vi "Launch Actors Wrapper.vi"() -> ()   [LabVIEW 2020]
uses:
  User Forms/TRExpRaw/TRExperimentsRaw.lvclass
  C:/Users/User/Desktop/Raman Program/Database OOP/source/Forms AF/Forms Controller/Form Controller/Panel Form Controller.lvclass
  Database OOP/Database Libraries/ADODB/ADODB Class/ADODB.lvclass
  C:/Users/User/Desktop/Raman Program/Database OOP/source/Database OOP/Database Libraries/Database Interfaces/Database Advanced Schema Class/Database Adv Schema.lvclass
  Database OOP/Database Libraries/ADODB/UDL Connection Class/UDL Connection.lvclass
  C:/Users/User/Desktop/Raman Program/Database OOP/source/Database OOP/Database Libraries/Database Interfaces/Database Connection Class/Database Connection.lvclass
  Forms Server/Form Server Wrapper/Form Server Wrapper.lvclass
  Database OOP/Table Libraries/Basic Table/Basic Table Class/Basic Table.lvclass
panel:
  in  "stop":bool
  out "Table Control":string[][](table)
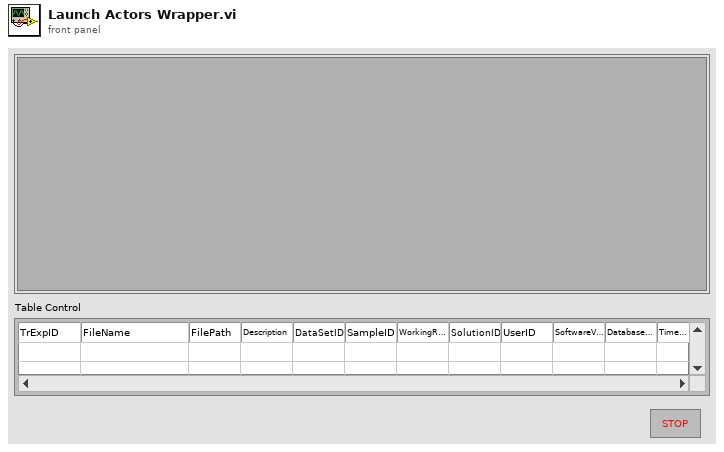
[diagram p1: front panel]
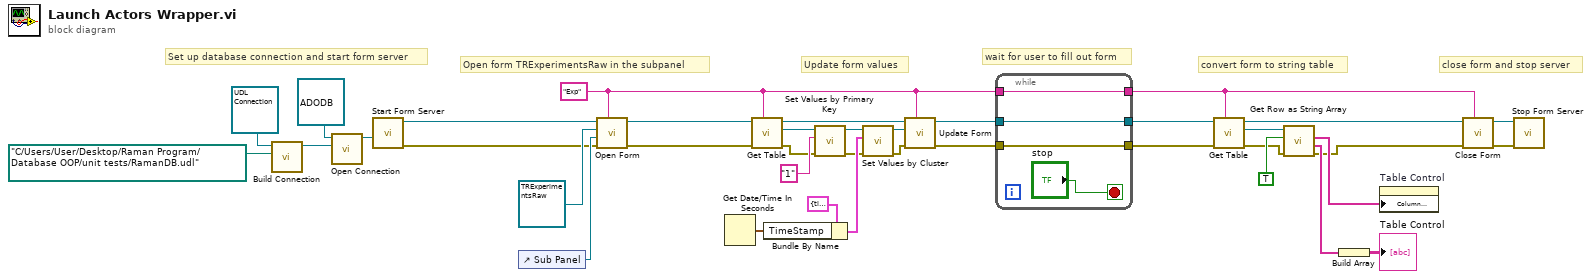
[diagram p0: block diagram]
diagram:
  w16 = "Exp" ("Name")
  # "close form and stop server"
  # "convert form to string table"
  # "wait for user to fill out form"
  # "Update form values"
  # "Open form TRExperimentsRaw in the subpanel"
  # "Set up database connection and start form server"
  n1 = call "Build Connection.vi"("*.udl file path"=path "C:/Users/User/Desktop/Raman Program/Database OOP/unit tests/RamanDB.udl", "UDL Connection in"=refnum<class "UDL Connection.lvclass"> refnum) -> ("UDL Connection out"=w27:refnum<class "UDL Connection.lvclass">)  [unwired: 8 in, 1 out]
  n2 = call-dynamic "Open Connection.vi"("Connection"=w27, "ADODB in"=refnum<class "ADODB.lvclass"> refnum ("ADODB.lvlib:ADODB.lvclass")) -> ("ADODB out"=w25:refnum<class "ADODB.lvclass">)  [unwired: 8 in, 1 out]
  n3 = call "Start Form Server.vi"("Database"=w25) -> ("error out"=w35:errorcluster, "Form Server Wrapper out"=w36:refnum<class "Form Server Wrapper.lvclass">)  [unwired: 9 in]
  n4 = control-ref of="Sub Panel"() -> (w38:refnum<vi>)
  n5 = call "Open Form.vi"("Name"=w16, "error in (no error)"=w35, "Sub Panel Refnum"=w38, "Form"=refnum<class "TRExperimentsRaw.lvclass"> refnum ("Forms.lvlib:TRExperimentsRaw.lvclass"), "Form Server Wrapper in"=w36) -> ("error out"=w30:errorcluster, "Form Server Wrapper out"=w34:refnum<class "Form Server Wrapper.lvclass">)  [unwired: 5 in]
  n6 = Get Date/Time In Seconds() -> (seconds since 1Jan1904=w21:timestamp)
  n7 = call "Get Table.vi"("Name"=w16, "error in (no error)"=w30, "Form Server Wrapper in"=w34) -> ("error out"=w8:errorcluster, "Table"=w19:refnum<class "Basic Table.lvclass">, "Form Server Wrapper out"=w33:refnum<class "Form Server Wrapper.lvclass">)  [unwired: 6 in]
  n8 = Bundle By Name(cluster=cluster{"TimeStamp":timestamp} {"TimeStamp"=timestamp(0 s since 1904-01-01)} ("input cluster"), "TimeStamp"=w21) -> (w22:cluster{"TimeStamp":timestamp})
  n9 = call "Set Values by Primary Key.vi"("error in (no error)"=w8, "Primary Key Value"="1", "Table in"=w19) -> ("error out"=w7:errorcluster, "Table out"=w23:refnum<class "Basic Table.lvclass">)  [unwired: 7 in]
  n10 = call "Set Values by Cluster.vi"("error in (no error)"=w7, "Cluster"=w22, "Table in"=w23) -> ("error out"=w6:errorcluster, "Table out"=w18:refnum<class "Basic Table.lvclass">)  [unwired: 7 in]
  n11 = call "Update Form.vi"("Name"=w16, "error in (no error)"=w6, "Table"=w18, "Form Server Wrapper in"=w33) -> ("error out"=w5:errorcluster, "Form Server Wrapper out"=w17:refnum<class "Form Server Wrapper.lvclass">)  [unwired: 6 in]
  n12 = while {
    tunnel: w17 -> [w42]
    tunnel: w16 -> [w41]
    tunnel: [w42] -> w15
    tunnel: [w41] -> w14
    tunnel: w5 -> [w39]
    tunnel: [w39] -> w4
    stop <- "stop" stop-if-true
  }
  n13 = call "Get Table.vi"("Name"=w14, "error in (no error)"=w4, "Form Server Wrapper in"=w15) -> ("error out"=w3:errorcluster, "Table"=w11:refnum<class "Basic Table.lvclass">, "Form Server Wrapper out"=w32:refnum<class "Form Server Wrapper.lvclass">)  [unwired: 6 in]
  n14 = call "Get Row as String Array.vi"("error in (no error)"=w3, "Keep DB Column Order (F)"=TRUE, "Table in"=w11) -> ("error out"=w2:errorcluster, "Row Values"=w13:string[], "Column Names"=w9:string[])  [unwired: 5 in, 1 out]
  n15 = Build Array(w13) -> (→"Table Control":string[][])
  n16 = property on="Table Control" class="Tbl (strict)"("Column Headers[]"=w9) -> ()  [unwired: 2 in, 2 out]
  n17 = call "Close Form.vi"("Name"=w14, "error in (no error)"=w2, "Form Server Wrapper in"=w32) -> ("error out"=w1:errorcluster, "Form Server Wrapper out"=w31:refnum<class "Form Server Wrapper.lvclass">)  [unwired: 7 in]
  n18 = call "Stop Form Server.vi"("error in (no error)"=w1, "Form Server Wrapper in"=w31) -> ()  [unwired: 9 in, 1 out]
